vi "FTW-SQLite-Core-Construct.vi"(0 "Database URI":string, 2 "Database Type":T1, 5 "Access Mode":T2, 11 "error in":errorcluster) -> (4 "SQLite Connection":refnum<data-value>, 6 "SQLite Version":string, 15 "error out":errorcluster)   [LabVIEW 2014]
uses:
  FTW-SQLite-Core-AccessMode.ctl
  FTW-SQLite-Core-DatabaseType.ctl
  FTW-SQLite-Core-Structure.ctl
  error/FTW-ERR-ThrowGenericError.vi
  error/FTW-ERR-ThrowError.vi
  error/FTW-ERR-NoErrorConstant.vi
  error/FTW-ERR-CallChain.vi
  string/FTW-STR-ReplaceWhitespace.vi
panel:
  # "Inputs"
  # "Outputs"
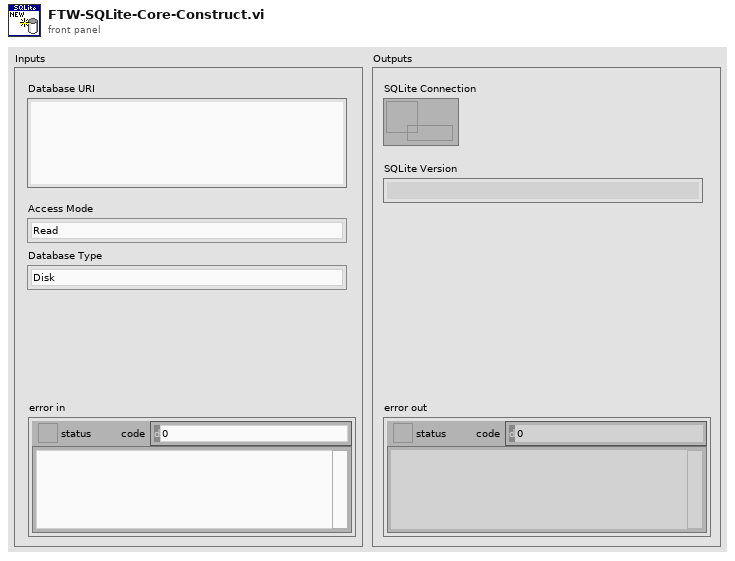
[diagram p1: front panel]
types:
  T1 = typedef "FTW-SQLite-Core-DatabaseType.ctl" = enum16{"Disk", "Memory"}
  T2 = typedef "FTW-SQLite-Core-AccessMode.ctl" = enum16{"Read", "Read/Write", "Read/Write/Create"}
  T3 = typedef "FTW-SQLite-Core-Structure.ctl" = cluster{"Connection":u64}
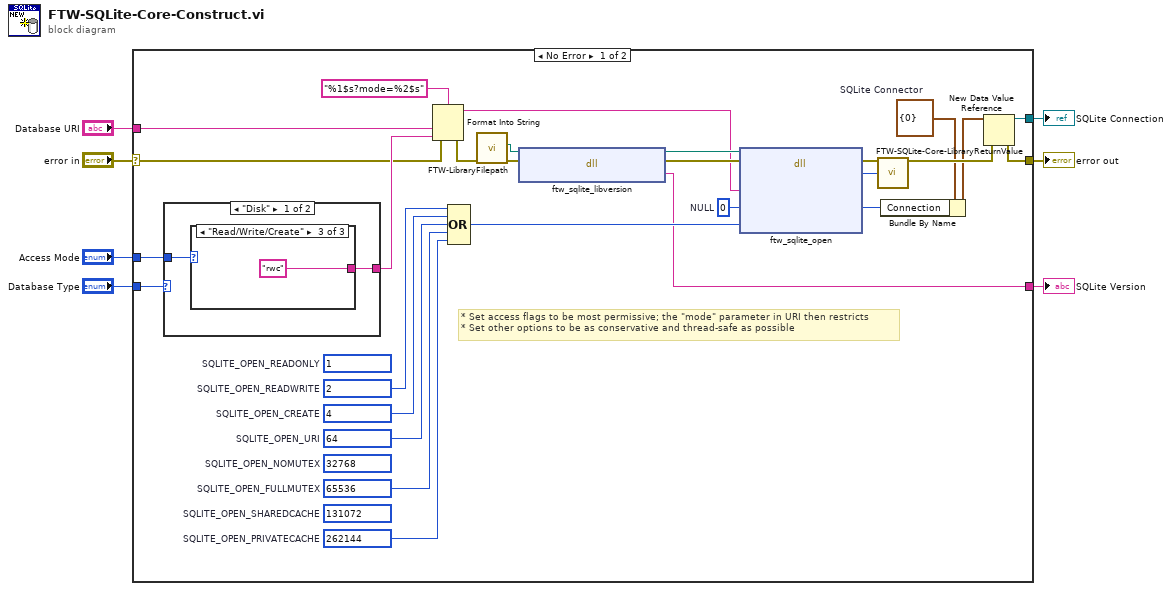
[diagram p0: block diagram]
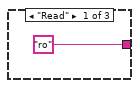
[diagram p2: hidden frame]
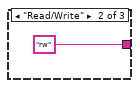
[diagram p3: hidden frame]
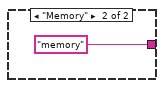
[diagram p4: hidden frame]
diagram:
  n1 = case shown="No Error" "error in" {
    selector: "error in" -> [w29 w42]
    tunnel: [w12 w42] -> w7
    tunnel: [w11 _] -> w1
    tunnel: [w18 _] -> w5
    tunnel: "Database URI" -> [w32 _]
    tunnel: "Access Mode" -> [w34 _]
    tunnel: "Database Type" -> [w23 _]
    frame No Error {
      w10 = T3 {"Connection"=0}  # SQLite Connector
      w14 = u64 0  # NULL
      w24 = u32 262144  # SQLITE_OPEN_PRIVATECACHE
      (unwired) u32 131072  # SQLITE_OPEN_SHAREDCACHE
      w25 = u32 65536  # SQLITE_OPEN_FULLMUTEX
      (unwired) u32 32768  # SQLITE_OPEN_NOMUTEX
      w26 = u32 64  # SQLITE_OPEN_URI
      w27 = u32 4  # SQLITE_OPEN_CREATE
      w28 = u32 2  # SQLITE_OPEN_READWRITE
      (unwired) u32 1  # SQLITE_OPEN_READONLY
      # "* Set access flags to be most permissive; the \"mode\" parameter in URI then restricts\n* Set other options to be as conservative and thread-safe as possible"
      n2 = case shown="\"Disk\"" w23 {
        tunnel: w34 -> [w37 _]
        tunnel: [w36 "memory"] -> w31
        frame "Disk" {
          n3 = case shown="\"Read/Write/Create\"" w37 {
            tunnel: ["ro" "rw" "rwc"] -> w36
            frame "Read" {
            }
            frame "Read/Write" {
            }
            frame "Read/Write/Create" {
            }
          }
        }
        frame "Memory" {
        }
      }
      n4 = Format Into String(format string="%1$s?mode=%2$s", error in=w29, w32, w31) -> (resulting string=w9:string, error out=w8:errorcluster)  [unwired: 1 in]
      n5 = Compound Arithmetic op=OR(w28, w27, w26, w25, w24) -> (w30:u32)
      n6 = call "FTW-LibraryFilepath.vi"("error in"=w8) -> ("error out"=w20:errorcluster, "Library Filepath"=w22:path)  [unwired: 8 in, 1 out]
      n7 = dll-call lib="?" fn="ftw_sqlite_libversion"(path in=w22, error in=w20) -> (path out=w21:path, error out=w19:errorcluster, "Return Value"=w18:string)  [unwired: 1 in]
      n8 = dll-call lib="?" fn="ftw_sqlite_open"(path in=w21, error in=w19, "Database URI"=w9, "Connection Handle"=w14, "Flags"=w30) -> (error out=w17:errorcluster, "Return Value"=w16:i32, "Connection Handle"=w15:u64)  [unwired: 3 in, 1 out]
      n9 = call "FTW-SQLite-Core-LibraryReturnValue.vi"("error in"=w17, "Return Value"=w16) -> ("error out"=w35:errorcluster)  [unwired: 13 in]
      n10 = Bundle By Name(cluster=w10, "Connection"=w15) -> (w13:T3)
      n11 = New Data Value Reference(data value=w13, error in=w35) -> (data value reference=w11:refnum<data-value>, error out=w12:errorcluster)
    }
    frame Error {
    }
  }
  "error out" <- w7
  "SQLite Version" <- w5
  "SQLite Connection" <- w1
